vi "make_axis_parallel_square_plane_coordinates.vi"(9 "Offset":sgl, 10 "Enum":enum16{"XY", "XZ", "YZ"}(ring), 11 "Min/Max":T1) -> (3 "appended array":cluster{"[0]":sgl, "[1]":sgl, "[2]":sgl}[](array[cluster]))   [LabVIEW 2020, in "3DPC_SurfacePlot.xctl"]
uses:
  <vilib>/Native 3D Graph/xcontrol/3DPC_SurfacePlot.xctl
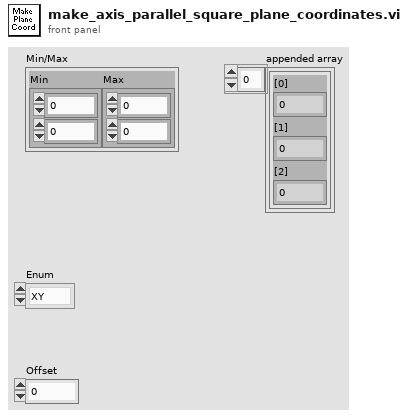
[diagram p1: front panel]
types:
  T1 = cluster{"Min":cluster{sgl, sgl}, "Max":cluster{sgl, sgl}}
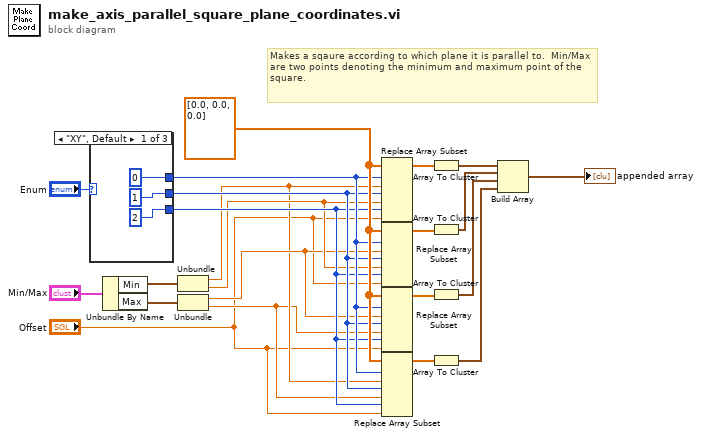
[diagram p0: block diagram]
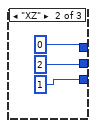
[diagram p2: hidden frame]
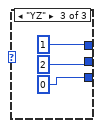
[diagram p3: hidden frame]
diagram:
  w18 = sgl[] [0.0, 0.0, 0.0]
  # "Makes a sqaure according to which plane it is parallel to.  Min/Max are two points denoting the minimum and maximum point of the square."
  n1 = case shown="\"XY\", Default" "Enum" {
    tunnel: [0 0 1] -> w17
    tunnel: [1 2 2] -> w16
    tunnel: [2 1 0] -> w15
    frame "XY", Default {
    }
    frame "XZ" {
    }
    frame "YZ" {
    }
  }
  n2 = Unbundle By Name("Min/Max") -> ("Min"=w20:cluster{sgl, sgl}, "Max"=w19:cluster{sgl, sgl})
  n3 = Unbundle(w20) -> (w12:sgl, w14:sgl)
  n4 = Unbundle(w19) -> (w13:sgl, w11:sgl)
  n5 = Replace Array Subset(array=w18, new element #1=w12, index #1=w17, new element #2=w14, index #2=w16, new element #3="Offset", index #3=w15) -> (w9:sgl[])
  n6 = Replace Array Subset(array=w18, new element #1=w13, index #1=w17, new element #2=w14, index #2=w16, new element #3="Offset", index #3=w15) -> (w8:sgl[])
  n7 = Replace Array Subset(array=w18, new element #1=w13, index #1=w17, new element #2=w11, index #2=w16, new element #3="Offset", index #3=w15) -> (w7:sgl[])
  n8 = Replace Array Subset(array=w18, new element #1=w12, index #1=w17, new element #2=w11, index #2=w16, new element #3="Offset", index #3=w15) -> (w6:sgl[])
  n9 = Array To Cluster(array=w9) -> (cluster=w5:cluster{"[0]":sgl, "[1]":sgl, "[2]":sgl})
  n10 = Array To Cluster(array=w8) -> (cluster=w4:cluster{"[0]":sgl, "[1]":sgl, "[2]":sgl})
  n11 = Array To Cluster(array=w7) -> (cluster=w3:cluster{"[0]":sgl, "[1]":sgl, "[2]":sgl})
  n12 = Array To Cluster(array=w6) -> (cluster=w2:cluster{"[0]":sgl, "[1]":sgl, "[2]":sgl})
  n13 = Build Array(w5, w4, w3, w2) -> (→"appended array":cluster{"[0]":sgl, "[1]":sgl, "[2]":sgl}[])
